vi "Write Stiffness Data.vi"(10 "Stiffness Data":cluster{"stiffnessCalculated":dbl[unit]} {"stiffnessCalculated" min=-888000000.0 max=888000000.0 format="%.2f"}, 11 "TestDataLog in":refnum<class "TestDataLog.lvclass">) -> (3 "TestDataLog out":refnum<class "TestDataLog.lvclass">)   [LabVIEW 2015, in "TestDataLog.lvclass"]
uses:
  TestDataLog.lvclass
  TestDataLog.lvclass/TestDataLog.ctl
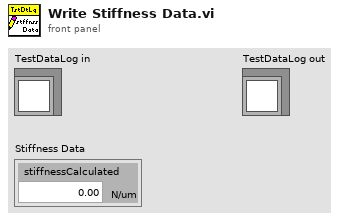
[diagram p1: front panel]
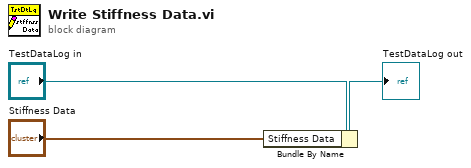
[diagram p0: block diagram]
diagram:
  n1 = Bundle By Name(cluster="TestDataLog in", "Stiffness Data"="Stiffness Data") -> (→"TestDataLog out":refnum<class "TestDataLog.lvclass">)
